vi "调试程序.vi"(9 "CAN端口":u16(ring) items=["0", "1"], 10 "设备索引号":u16(ring) items=["0", "1", "2", "3", "4", "5", "6", "7", "8", "9", "10", "11", "12", "13", "14", "15", ""], 11 "CAN卡类型":u16(ring)=4 items=["PCI5121"=1, "PCI9810"=2, "USBCAN1"=3, "USBCAN2"=4, "PCI9820"=5, "CAN232"=6, "PCI5110"=7, "CANLite(mini)"=8, "ISA9620"=9, "ISA5420"=10, "PC104CAN"=11, "CANETE"=12, "DNP9810"=13]) -> ()   [LabVIEW 2013]
uses:
  <vilib>/Utility/file.llb/Write To Spreadsheet File (string).vi
panel:
  in  "帧2":bool=TRUE
  in  "帧1":bool=TRUE
  in  "Conversion":enum16{"HEX_Conversion", "Decimal_Conversion"}(ring)
  in  "123":T1
  in  "保存数据":bool
  out "发送成功":bool
  in  "开始":bool
  in  "设定刷新条数":i32=10000 caption="Set_Refresh_Num"
  out "Num Rows":u32
  out "VCI_CAN_OBJ_R":T2={"ID"=0, "TimeStamp"=0, "TimeFlag"=0, "SendType"=1, "RemoteFlag"=0, "ExternFlag"=0, "DataLen"=8, 0, 0, 0, 0, 0, 0, 0, 0, 0, 0, 0}
  out "VCI_CAN_OBJ_T":T2={"ID"=0, "TimeStamp"=0, "TimeFlag"=0, "SendType"=1, "RemoteFlag"=0, "ExternFlag"=0, "DataLen"=8, 0, 0, 0, 0, 0, 0, 0, 0, 0, 0, 0}
  in  "停止":bool
  out "Multicolumn Listbox":i32(listbox)
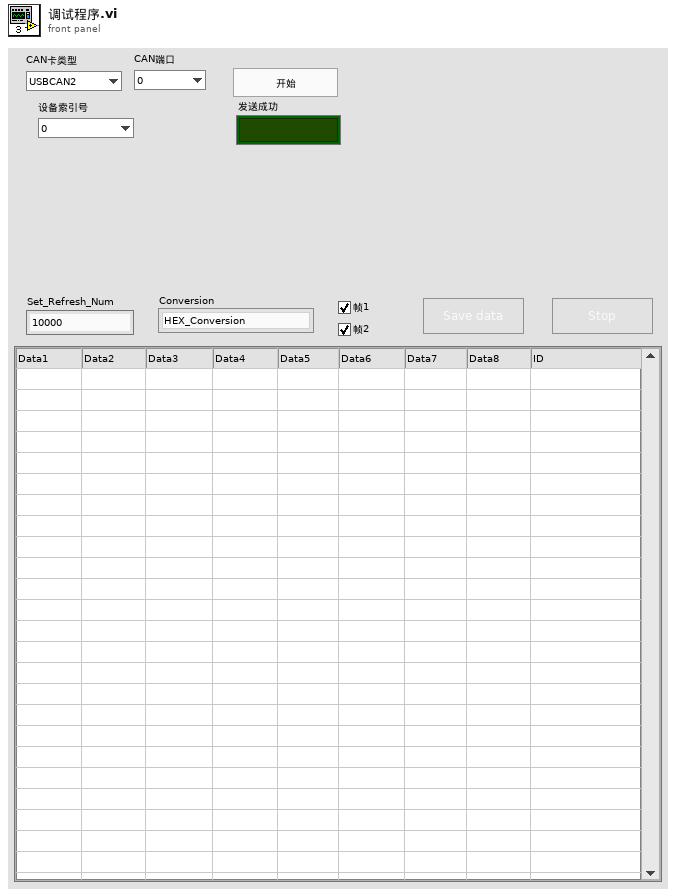
[diagram p1: front panel]
types:
  T1 = cluster{"ID":u32, "TimeStamp":u32, "TimeFlag":u8, "SendType":u8, "RemoteFlag":u8, "ExternFlag":u8, "DataLen":u8, "1":u8, "2":u8, "3":u8, "4":u8, "5":u8, "6":u8, "7":u8, "8":u8, "9":u8, "10":u8, "11":u8}
  T2 = cluster{"ID":u32, "TimeStamp":u32, "TimeFlag":u8, "SendType":u8, "RemoteFlag":u8, "ExternFlag":u8, "DataLen":u8, u8, u8, u8, u8, u8, u8, u8, u8, u8, u8, u8}
  T3 = enum32{"Invalid", "Standard", "Closed", "Hidden", "Minimized", "Maximized"}
  T4 = cluster{"return type":u32, "pReceive":cluster{"ID":u32, "TimeStamp":u32, "TimeFlag":u8, "SendType":u8, "RemoteFlag":u8, "ExternFlag":u8, "DataLen":u8, "1":u8, "2":u8, "3":u8, "4":u8, "5":u8, "6":u8, "7":u8, "8":u8, "9":u8, "10":u8, "11":u8}[]}
  T5 = cluster{"ID":u32, "TimeStamp":u32, "TimeFlag":u8, "SendType":u8, "RemoteFlag":u8, "ExternFlag":u8, "DataLen":u8, "1":u8, "2":u8, "3":u8, "4":u8, "5":u8, "6":u8, "7":u8, "8":u8, "9":u8, "10":u8, "11":u8}[]
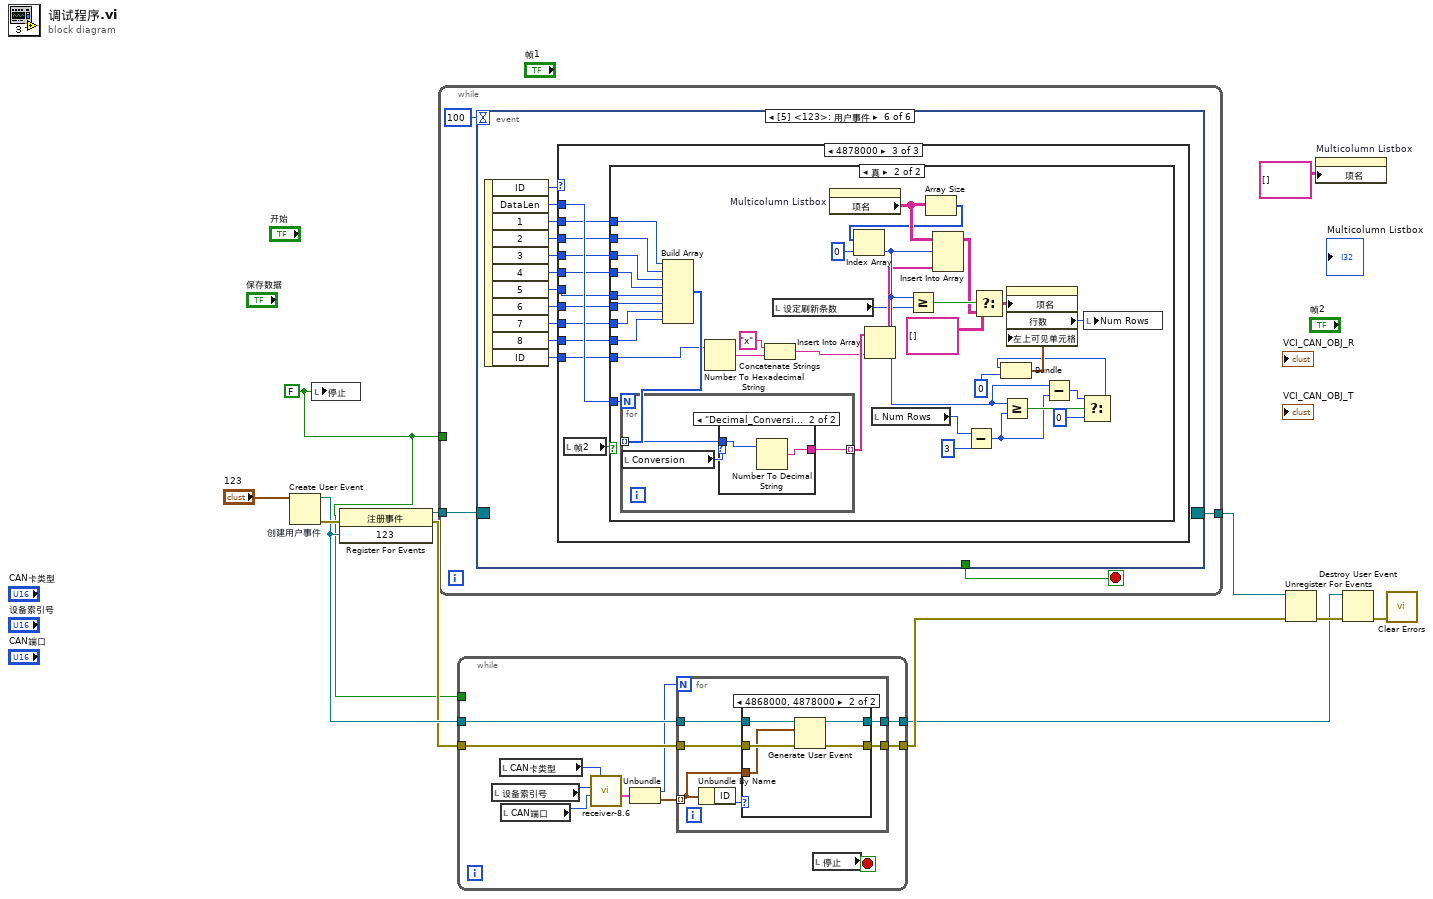
[diagram p0: block diagram]
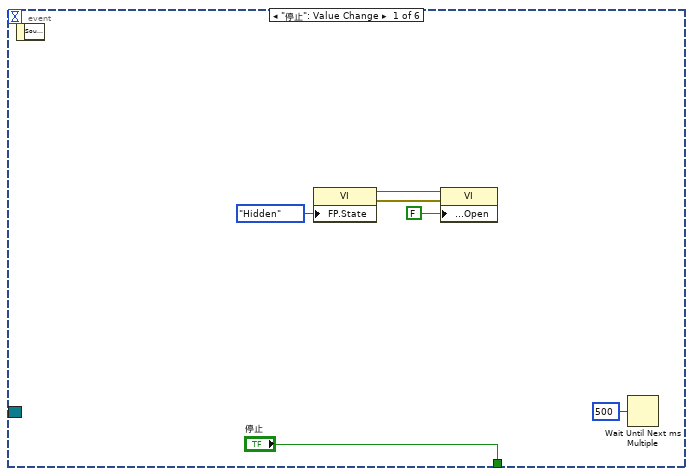
[diagram p3: hidden frame]
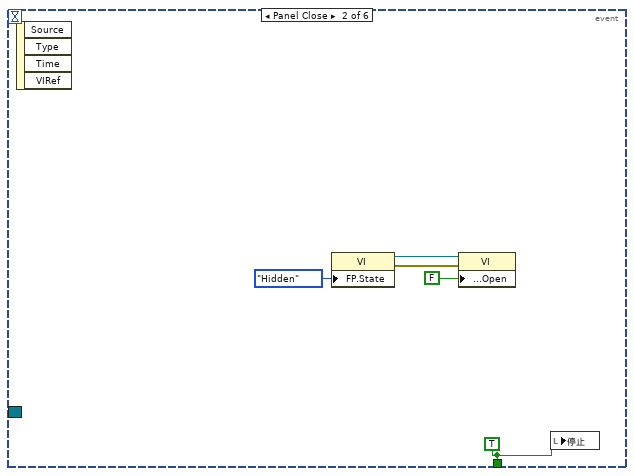
[diagram p4: hidden frame]
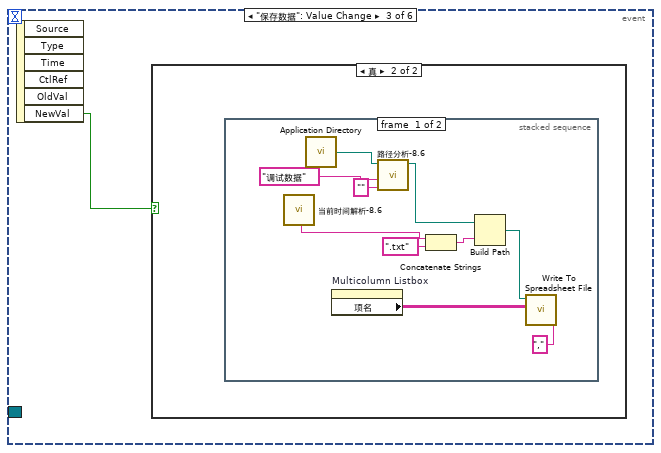
[diagram p5: hidden frame]
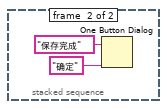
[diagram p7: hidden frame]
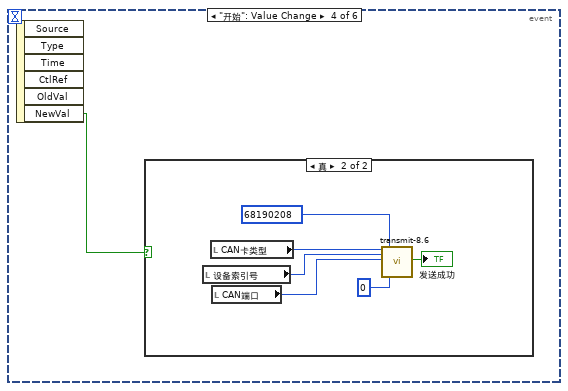
[diagram p8: hidden frame]
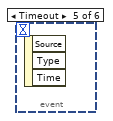
[diagram p10: hidden frame]
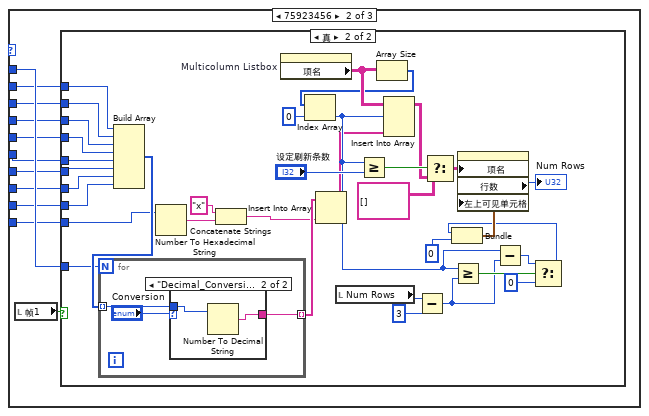
[diagram p12: hidden frame]
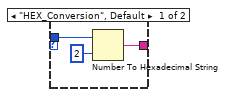
[diagram p14: hidden frame]
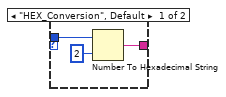
[diagram p16: hidden frame]
diagram:
  w1 = FALSE ("stop")
  n1 = Create User Event "创建用户事件"(user event datatype="123") -> (user event=w7:refnum<user-event>, error out=w11:errorcluster)  [unwired: 1 in]
  n2 = local write "停止"(w1) -> ()
  n3 = register-events(error in=w11, w7) -> (reference out=w9:refnum<event-registration>, error out=w6:errorcluster)  [unwired: 1 in]
  n4 = while {
    tunnel: w9 -> [w13]
    tunnel: [w16] -> w8
    tunnel: w1 -> [_]
    stop <- w14 stop-if-true
    n5 = event shown="[5] <123>: 用户事件" {
      selector: w13 -> [_ _ _ _ _ _]
      dyn-events: [_ _ _ _ _ _] -> w16
      timeout: 100 -> [_ _ _ _ _ _]
      tunnel: ["停止" w27 _ _ _ _] -> w14
      event "停止": Value Change {
        n6 = event-data() -> ()  [unwired: 1 in, 1 out]
        n7 = property class="VI"("FP.State"=T3."Hidden" ("前面板窗口:状态")) -> (reference out=w19:refnum<vi>, error out=w20:errorcluster)  [unwired: 2 in]
        n8 = property class="VI"(reference=w19, error in=w20, "Front Panel.Open"=FALSE ("前面板窗口:打开")) -> ()  [unwired: 2 out]
        n9 = Wait Until Next ms Multiple(millisecond multiple=u32 500 ("毫秒倍数")) -> ()  [unwired: 1 out]
      }
      event Panel Close {
        w27 = TRUE ("stop")
        n10 = event-data() -> ()  [unwired: 1 in, 4 out]
        n11 = property class="VI"("FP.State"=T3."Hidden" ("前面板窗口:状态")) -> (reference out=w25:refnum<vi>, error out=w26:errorcluster)  [unwired: 2 in]
        n12 = property class="VI"(reference=w25, error in=w26, "Front Panel.Open"=FALSE ("前面板窗口:打开")) -> ()  [unwired: 2 out]
        n13 = local write "停止"(w27) -> ()
      }
      event "保存数据": Value Change {
        n14 = event-data() -> ("NewVal"=w28:bool)  [unwired: 1 in, 5 out]
        n15 = case shown="真" w28 {
          frame False {
          }
          frame True {
            n16 = stacked-sequence {
              frame #0 {
                n17 = call "当前时间解析-8.6.vi"() -> ("名称格式时间"=w29:string)  [unwired: 10 in, 9 out]
                n18 = call <vilib>:"Application Directory.vi"() -> ("Application Directory"=w31:path)
                n19 = property on="Multicolumn Listbox" class="MCListbox (严格)"() -> ("项名"=w38:string[][])  [unwired: 2 in, 2 out]
                n20 = call "路径分析-8.6.vi"("第二个文件夹"="", "第一个文件夹"="调试数据" ("名称或相对路径"), "输入路径"=w31) -> ("输出路径"=w32:path)  [unwired: 8 in]
                n21 = Concatenate Strings(w29, ".txt" ("字符串")) -> (w35:string)
                n22 = Build Path(base path=w32, name or relative path=w35) -> (appended path=w34:path)
                n23 = call-poly <vilib>:"Write To Spreadsheet File.vi"("delimiter (\\t)"="," ("delimiter (\\t)"), "2D data"=w38, "file path (dialog if empty)"=w34) -> ()  [unwired: 5 in, 1 out]
              }
              frame #1 {
                n24 = One Button Dialog(message="保存完成" ("消息"), button name ("OK")="确定" ("按钮名称（“确定”）")) -> ()  [unwired: 1 out]
              }
            }
          }
        }
      }
      event "开始": Value Change {
        n25 = event-data() -> ("NewVal"=w41:bool)  [unwired: 1 in, 5 out]
        n26 = case shown="真" w41 {
          frame False {
          }
          frame True {
            n27 = local read "设备索引号"() -> (w45:u16)
            n28 = local read "CAN卡类型"() -> (w46:u16)
            n29 = local read "CAN端口"() -> (w44:u16)
            n30 = call "transmit-8.6.vi"("can卡类型"=w46, "设备索引号"=w45, "CAN端口"=w44, "ID"=u32 68190208, "SendType"=u8 0) -> ("发送成功"=→"发送成功":bool)  [unwired: 11 in, 3 out]
          }
        }
      }
      event Timeout {
        n31 = event-data() -> ()  [unwired: 1 in, 3 out]
      }
      event User Event {
        n32 = event-data() -> ("ID"=w48:u32, "DataLen"=w58:u8, "1"=w57:u8, "2"=w56:u8, "3"=w55:u8, "4"=w54:u8, "5"=w53:u8, "6"=w52:u8, "7"=w51:u8, "8"=w50:u8, "ID"=w49:u32)  [unwired: 1 in]
        n33 = case shown="4878000" w48 {
          tunnel: w58 -> [_ w69 w123]
          tunnel: w57 -> [_ w68 w122]
          tunnel: w56 -> [_ w67 w121]
          tunnel: w55 -> [_ w66 w120]
          tunnel: w54 -> [_ w65 w119]
          tunnel: w53 -> [_ w64 w118]
          tunnel: w52 -> [_ w63 w117]
          tunnel: w51 -> [_ w62 w116]
          tunnel: w50 -> [_ w61 w115]
          tunnel: w49 -> [_ w60 w114]
          frame 0, Default {
          }
          frame 75923456 {
            n34 = local read "帧1"() -> (w59:bool)
            n35 = case shown="真" w59 {
              tunnel: w69 -> [_ w84]
              tunnel: w68 -> [_ w83]
              tunnel: w67 -> [_ w82]
              tunnel: w66 -> [_ w81]
              tunnel: w65 -> [_ w80]
              tunnel: w64 -> [_ w79]
              tunnel: w63 -> [_ w78]
              tunnel: w62 -> [_ w77]
              tunnel: w61 -> [_ w76]
              tunnel: w60 -> [_ w75]
              frame False {
              }
              frame True {
                n36 = Build Array(w83, w82, w81, w80, w79, w78, w77, w76) -> (w101:u8[])
                n37 = for {
                  N: w84 -> [_]
                  tunnel: w101 -> [w107] mode=indexing
                  tunnel: [w106] -> w71 mode=indexing
                  n38 = case shown="\"Decimal_Conversion\"" "Conversion" {
                    tunnel: w107 -> [w109 w111]
                    tunnel: [w108 w112] -> w106
                    frame "HEX_Conversion", Default {
                      n39 = Number To Hexadecimal String(1:i16 2 ("width (-)"), 2:w109) -> (0:w108:string)
                    }
                    frame "Decimal_Conversion" {
                      n40 = Number To Decimal String(number=w111) -> (decimal integer string=w112:string)  [unwired: 1 in]
                    }
                  }
                }
                n41 = Number To Hexadecimal String(2:w75) -> (0:w74:string)  [unwired: 1 in]
                n42 = Concatenate Strings("x" ("字符串"), w74) -> (w70:string)
                n43 = property on="Multicolumn Listbox" class="MCListbox (严格)"() -> ("项名"=w103:string[][])  [unwired: 2 in, 2 out]
                n44 = Insert Into Array(array=w71, new element=w70) -> (w72:string[])  [unwired: 1 in]
                n45 = local read "Num Rows"() -> (w89:u32)
                n46 = Array Size(array=w103) -> (size(s)=w102:i32[])
                n47 = Index Array(array=w102, index=0) -> (element=w88:i32)
                n48 = Greater Or Equal?(x=w88, y="设定刷新条数") -> (x >= y?=w100:bool)
                n49 = Insert Into Array(array=w103, index (row)=w88, new element=w72) -> (w98:string[][])  [unwired: 1 in]
                n50 = Subtract(x=w89, y=u32 3) -> (x-y=w91:u32)
                n51 = Select(t=string[][] [], s=w100, f=w98) -> (s? t:f=w99:string[][])
                n52 = Greater Or Equal?(x=w88, y=w91) -> (x >= y?=w92:bool)
                n53 = Subtract(x=w88, y=w91) -> (x-y=w87:u32)
                n54 = Select(t=w87, s=w92, f=u32 0) -> (s? t:f=w85:u32)
                n55 = Bundle("f"=w85, 0) -> (w93:cluster{"f":u32, i32})  [unwired: 1 in]
                n56 = property on="Multicolumn Listbox" class="MCListbox (严格)"("项名"=w99, "左上可见单元格"=w93) -> ("行数"=→"Num Rows":u32)  [unwired: 2 in, 2 out]
              }
            }
          }
          frame 75988992 {
            n57 = local read "帧2"() -> (w113:bool)
            n58 = case shown="真" w113 {
              tunnel: w123 -> [_ w141]
              tunnel: w122 -> [_ w140]
              tunnel: w121 -> [_ w139]
              tunnel: w120 -> [_ w138]
              tunnel: w119 -> [_ w137]
              tunnel: w118 -> [_ w136]
              tunnel: w117 -> [_ w135]
              tunnel: w116 -> [_ w134]
              tunnel: w115 -> [_ w133]
              tunnel: w114 -> [_ w132]
              frame False {
              }
              frame True {
                n59 = Build Array(w140, w139, w138, w137, w136, w135, w134, w133) -> (w155:u8[])
                n60 = for {
                  N: w141 -> [_]
                  tunnel: w155 -> [w161] mode=indexing
                  tunnel: [w160] -> w128 mode=indexing
                  n61 = local read "Conversion"() -> (w159:enum16{"HEX_Conversion", "Decimal_Conversion"})
                  n62 = case shown="\"Decimal_Conversion\"" w159 {
                    tunnel: w161 -> [w163 w165]
                    tunnel: [w162 w166] -> w160
                    frame "HEX_Conversion", Default {
                      n63 = Number To Hexadecimal String(1:i16 2 ("width (-)"), 2:w163) -> (0:w162:string)
                    }
                    frame "Decimal_Conversion" {
                      n64 = Number To Decimal String(number=w165) -> (decimal integer string=w166:string)  [unwired: 1 in]
                    }
                  }
                }
                n65 = Number To Hexadecimal String(2:w132) -> (0:w131:string)  [unwired: 1 in]
                n66 = Concatenate Strings("x" ("字符串"), w131) -> (w127:string)
                n67 = local read "设定刷新条数"() -> (w124:i32)
                n68 = property on="Multicolumn Listbox" class="MCListbox (严格)"() -> ("项名"=w157:string[][])  [unwired: 2 in, 2 out]
                n69 = Insert Into Array(array=w128, new element=w127) -> (w129:string[])  [unwired: 1 in]
                n70 = local read "Num Rows"() -> (w125:u32)
                n71 = Array Size(array=w157) -> (size(s)=w156:i32[])
                n72 = Index Array(array=w156, index=0) -> (element=w145:i32)
                n73 = Greater Or Equal?(x=w145, y=w124) -> (x >= y?=w154:bool)
                n74 = Insert Into Array(array=w157, index (row)=w145, new element=w129) -> (w152:string[][])  [unwired: 1 in]
                n75 = Subtract(x=w125, y=u32 3) -> (x-y=w147:u32)
                n76 = Select(t=string[][] [], s=w154, f=w152) -> (s? t:f=w153:string[][])
                n77 = Greater Or Equal?(x=w145, y=w147) -> (x >= y?=w148:bool)
                n78 = Subtract(x=w145, y=w147) -> (x-y=w144:u32)
                n79 = Select(t=w144, s=w148, f=u32 0) -> (s? t:f=w142:u32)
                n80 = Bundle("f"=w142, 0) -> (w149:cluster{"f":u32, i32})  [unwired: 1 in]
                n81 = property on="Multicolumn Listbox" class="MCListbox (严格)"("项名"=w153, "左上可见单元格"=w149) -> ("行数"=w126:u32)  [unwired: 2 in, 2 out]
                n82 = local write "Num Rows"(w126) -> ()
              }
            }
          }
        }
      }
    }
  }
  n83 = while {
    tunnel: w7 -> [w177]
    tunnel: w6 -> [w176]
    tunnel: [w175] -> w4
    tunnel: [w174] -> w5
    tunnel: w1 -> [_]
    stop <- w173 stop-if-true
    n84 = local read "设备索引号"() -> (w171:u16)
    n85 = local read "CAN卡类型"() -> (w172:u16)
    n86 = local read "CAN端口"() -> (w170:u16)
    n87 = call "receiver-8.6.vi"("CAN端口"=w170, "设备索引号"=w171, "CAN卡类型"=w172) -> ("输出簇"=w169:T4)  [unwired: 1 in, 5 out]
    n88 = Unbundle(w169) -> ("return type"=w168:u32, "pReceive"=w167:T5)
    n89 = for {
      N: w168 -> [_]
      tunnel: w177 -> [w183]
      tunnel: w176 -> [w182]
      tunnel: [w181] -> w175
      tunnel: [w180] -> w174
      tunnel: w167 -> [w178] mode=indexing
      n90 = Unbundle By Name(w178) -> ("ID"=w179:u32)
      n91 = case shown="4868000, 4878000" w179 {
        tunnel: w183 -> [w185 w190]
        tunnel: w182 -> [w184 w189]
        tunnel: [w185 w188] -> w181
        tunnel: [w184 w187] -> w180
        tunnel: w178 -> [_ w186]
        frame 0, Default {
        }
        frame 75923456, 75988992 {
          n92 = Generate User Event(user event=w190, event data cluster=w186, error in=w189) -> (user event out=w188:refnum<user-event>, error out=w187:errorcluster)  [unwired: 1 in]
        }
      }
    }
    n93 = local read "停止"() -> (w173:bool)
  }
  n94 = Unregister For Events(event registration refnum=w8, error in=w5) -> (error out=w10:errorcluster)
  n95 = property on="Multicolumn Listbox" class="MCListbox (严格)"("项名"=string[][] [] ("Item Names")) -> ()  [unwired: 2 in, 2 out]
  n96 = Destroy User Event(user event=w4, error in=w10) -> (error out=w2:errorcluster)
  n97 = call <vilib>:"Clear Errors.vi"("error in (no error)"=w2) -> ()  [unwired: 6 in, 1 out]
